vi "13_2.vi"() -> ()   [LabVIEW 2018]
panel:
  out "Numeric":dbl=1106724616194525.0
  in  "Input":string="1000052\n23,x,x,x,x,x,x,x,x,x,x,x,x,x,x,x,x,37,x,x,x,x,x,863,x,x,x,x,x,x,x,x,x,x,x,19,13,x,x,x,17,x,x,x,x,x,x,x,x,x,x,x,29,x,571,x,x,x,x,x,x,x,x,x,x,x,x,x,x,x,x,x,x,x,x,x,x,x,x,x,x,x,x,x,x,x,x,x,x,x,x,x,x,x,x,41"
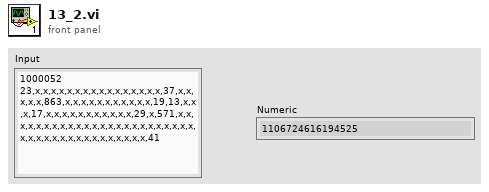
[diagram p1: front panel]
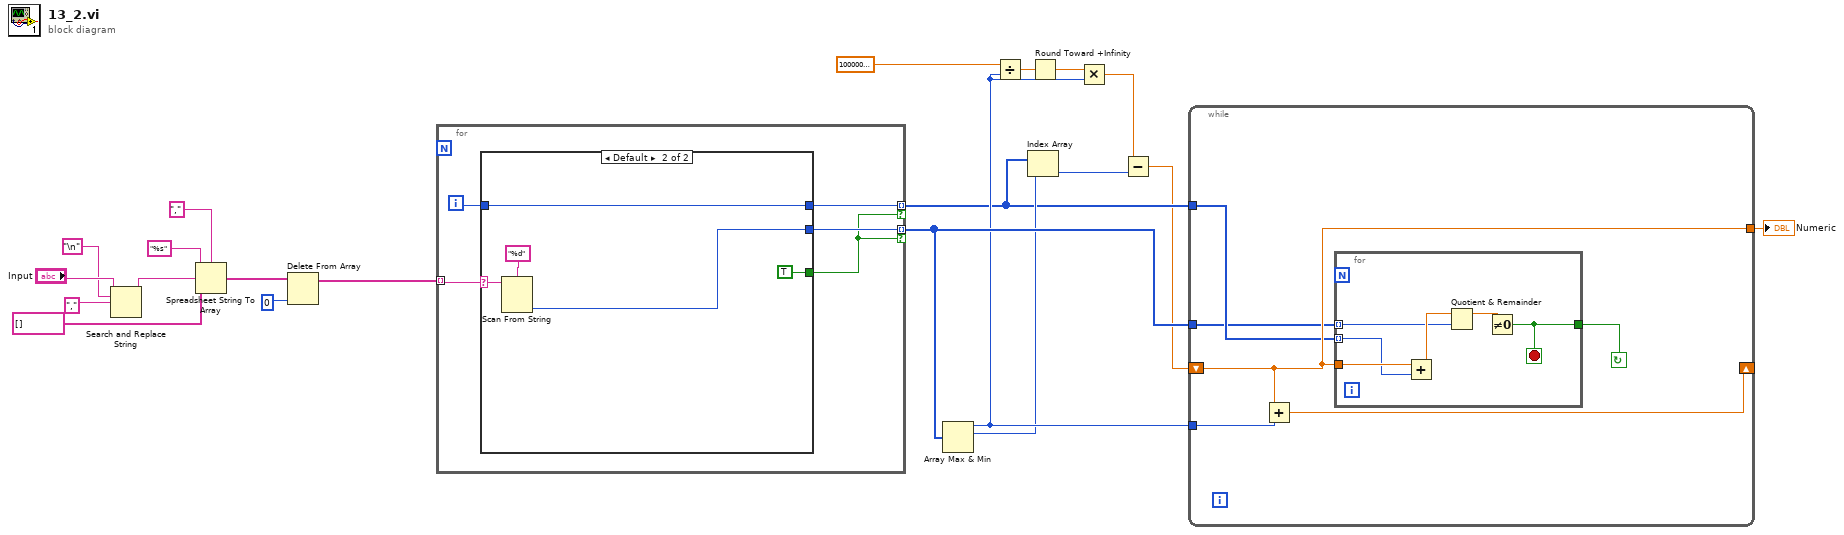
[diagram p0: block diagram]
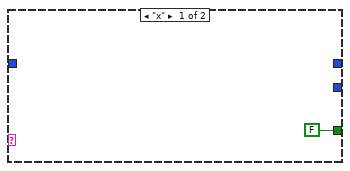
[diagram p2: hidden frame]
diagram:
  n1 = Search and Replace String(input string="Input", search string="\n", replace string=",") -> (result string=w17:string)  [unwired: 5 in, 3 out]
  n2 = Spreadsheet String To Array(delimiter (Tab)=",", format string="%s", spreadsheet string=w17, array type (2D Dbl)=string[] []) -> (array=w14:string[])
  n3 = Delete From Array(array=w14, index=0) -> (array with subset deleted=w12:string[])  [unwired: 1 in, 1 out]
  n4 = for {
    tunnel: w12 -> [w26] mode=indexing
    tunnel: [w24] -> w7 mode=indexing if=w22
    tunnel: [w23] -> w4 mode=indexing if=w22
    i -> [w25]
    n5 = case shown="Default" w26 {
      selector: w26 -> [_ w31]
      tunnel: [FALSE TRUE] -> w22
      tunnel: w25 -> [_ w28]
      tunnel: [_ w29] -> w24
      tunnel: [_ w28] -> w23
      frame "x" {
      }
      frame Default {
        n6 = Scan From String(format string="%d", input string=w31) -> (output 1=w29:i32)  [unwired: 3 in, 3 out]
      }
    }
  }
  n7 = Array Max & Min(array=w7) -> (max value=w6:i32, max index (indices)=w5:i32)  [unwired: 2 out]
  n8 = Divide(x=100000000000000.0, y=w6) -> (x/y=w10:dbl)
  n9 = Index Array(array=w4, index=w5) -> (element=w3:i32)
  n10 = Round Toward +Infinity(x=w10) -> (ceil(x): smallest int >= x=w9:dbl)
  n11 = Multiply(x=w9, y=w6) -> (x*y=w2:dbl)
  n12 = Subtract(x=w2, y=w3) -> (x-y=w1:dbl)
  n13 = while {
    tunnel: [w37] -> w11
    shift-right: [w36] -> _
    shift-left: w1 -> [w37]
    tunnel: w6 -> [w33]
    tunnel: w4 -> [w35]
    tunnel: w7 -> [w34]
    stop <- w38 continue-if-true
    n14 = Add(x=w37, y=w33) -> (x+y=w36:dbl)
    n15 = for {
      tunnel: w37 -> [w44]
      tunnel: [w42] -> w38
      tunnel: w35 -> [w40] mode=indexing
      tunnel: w34 -> [w39] mode=indexing
      stop <- w42 stop-if-true
      n16 = Add(x=w44, y=w40) -> (x+y=w43:dbl)
      n17 = Quotient & Remainder(x=w43, y=w39) -> (x-y*floor(x/y)=w41:dbl)  [unwired: 1 out]
      n18 = Not Equal To 0?(x=w41) -> (x != 0?=w42:bool)
    }
  }
  "Numeric" <- w11
